vi "PH_Timing.PC Timing Mode.vi"(0 "i ref in":refnum<vi>, 2 "Timing Mode":T1 {"T2" min=0 max=6000 step=2}, 5 "error IO":errorcluster) -> (14 "i ref out":refnum<vi>, 19 "error out":errorcluster)   [LabVIEW 2014, in "PH_Timing.lvlib"]
doc: "This is a certain process case of Timing."
uses:
  PH_Timing.lvlib
  PH_Timing.Timing Mode.ctl
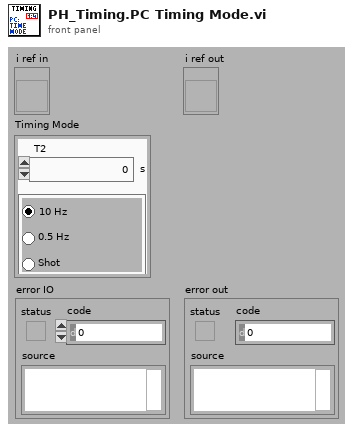
[diagram p1: front panel]
types:
  T1 = typedef "PH_Timing.lvlib/PH_Timing.Timing Mode.ctl" = cluster{"T2":i16, "Modeselector":enum32{"10 Hz", "0.5 Hz", "Shot"}}
  T2 = typedef "PH_Timing.lvlib/PH_Timing.i attribute.ctl" = cluster{"Sequencer":cluster{"linked?":bool, "Proc State":string, "Ref State":refnum<vi>}, "Gate Generator":cluster{"GD":cluster{"Device Status":T3, "linked?":bool}, "Settings":T4, "GUI Ref":refnum<vi>}, "Interlock Bypass":cluster{"Instancename":string, "Switch linked?":bool, "Device Status":T3, "Ref Status":refnum<vi>}, "Roughtuner":cluster{"Settings":T5, "GUI Ref":refnum<vi>, "GD":cluster{"Device Status":T3, "linked?":bool}}, "0,5Hz Gater":cluster{"Settings":T6, "GUI Ref":refnum<vi>, "GD":cluster{"Device Status":T3, "linked?":bool}}, "Slow Trigger":cluster{"Settings":T7, "GUI Ref":refnum<vi>, "Service ID Delay":i32, "Service ID Ext Trig":i32, "Wanted Settings":T7}, "Timing Mode":cluster{"Mode":T1, "GUI Ref":refnum<vi>, "Service ID T2":i32, "Service ID Mode":i32, "Wanted Mode":T1}, "ns Generator":cluster{"Settings":T8, "ns Generator Settings":refnum<vi>, "GD":cluster{"Device Status":T3, "linked?":bool}}, "Phase FEs":cluster{"Settings":T11, "GUI Ref":refnum<vi>, "Service ID Phase":i32, "Wanted Settings":T11}, "GD GUI Refs":refnum<vi>[], "Heads":T12[], "GUI Ref Delete":refnum<vi>}
  T3 = typedef "PH_StatusHandler.lvlib/PH_StatusHandler.Status.ctl" = i16
  T4 = typedef "PH_Timing.lvlib/PH_Timing.GateGen.ctl" = cluster{"Instance":string, "Channel Gate":i32, "Channel T2":i32, "Width Gate":dbl, "Width T2":dbl, "Delay Gate":dbl, "Delay T2":dbl, "Gate activ":bool, "T2 activ":bool, "System Mode":enum16{"Normal", "Single", "Burst", "Duty Cycle"}}
  T5 = typedef "PH_Timing.lvlib/PH_Timing.Roughtuner.ctl" = cluster{"Instance":string, "Phase PHELIX / UNILAC":cluster{"Channel":u16, "relative to":u16, "Delay [ms]":dbl}, "Pulse Length":cluster{"Channel":u16, "relative to":u16, "Delay [ms]":dbl}, "Trigger":cluster{"externally?":bool, "Rate [Hz]":dbl}}
  T6 = typedef "PH_Timing.lvlib/PH_Timing.0.5HzGater.ctl" = cluster{"Instance":string, "Channel ns FE Delay":i32, "Channel 0.5Hz":i32, "Width ns FE Delay":dbl, "Width 0.5Hz":dbl, "Delay ns FE Delay":dbl, "Delay 0.5Hz":dbl, "ns FE Delay active":bool, "0.5Hz activ":bool, "ns FE Delay inverted":bool, "0.5Hz inverted":bool}
  T7 = typedef "PH_Timing.lvlib/PH_Timing.Slow Trigger Settings.ctl" = cluster{"Delay":dbl, "externally triggered?":bool}
  T8 = typedef "PH_Timing.lvlib/PH_Timing.ns Generator.ctl" = cluster{"Instance":string, "Phase fs / ns FE":cluster{"Channel":T9, "Settings":T10}}
  T9 = typedef "Stanford Research DG645 - Driver.lvlib/Channel.ctl" = i32
  T10 = typedef "PH_SRDG645.lvlib/PH_SRDG645.Channel Settings.ctl" = cluster{"Delay [s]":dbl, "relative to":i32}
  T11 = typedef "PH_Timing.lvlib/PH_Timing.Phase FEs.ctl" = cluster{"Phase":dbl}
  T12 = typedef "PH_Timing.lvlib/PH_Timing.PU Data.ctl" = cluster{"linked?":bool, "Data":T13, "GD":cluster{"Device Status":T3, "linked?":bool}, "GUI Ref":refnum<vi>, "PU":T14}
  T13 = typedef "PH_Timing.lvlib/PH_Timing.PU Info.ctl" = cluster{"Act CH?":bool, "GD":string, "CH":i32, "Delay":dbl, "active":bool, "in Use?":bool}
  T14 = typedef "PH_PP_Common.lvlib/PH_PP_Common.PUs.ctl" = enum16{"no Info", "PA-19mm-1", "PA-19mm-2", "PA-45mm-PILC", "PA-45mm-MAIN", "MA-PU-1", "MA-PU-2", "MA-PU-3", "MA-PU-4", "MA-PU-5", "MA-PU-6", "MA-FR", "MA-PILC", "PA-45mm-DP"}
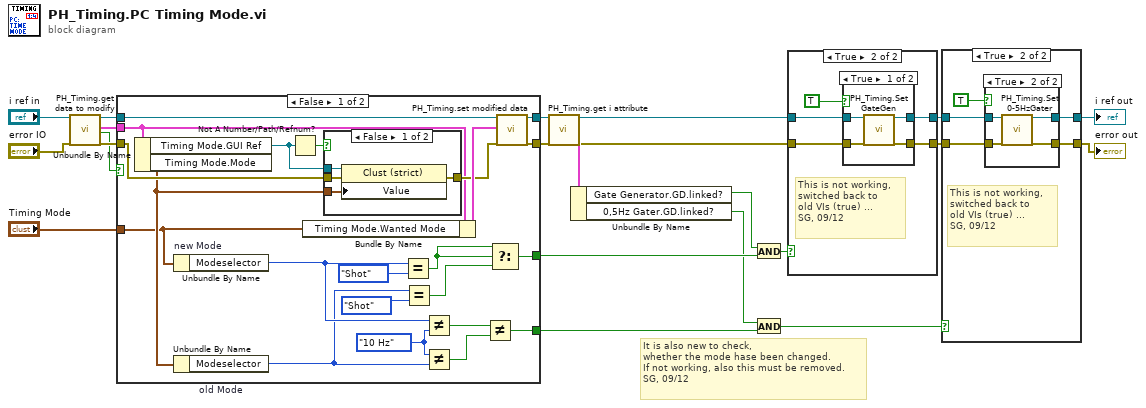
[diagram p0: block diagram]
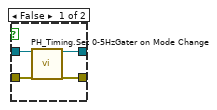
[diagram p3: hidden frame]
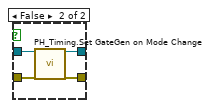
[diagram p5: hidden frame]
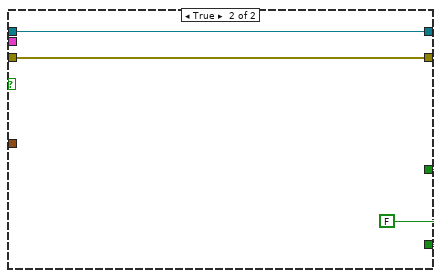
[diagram p7: hidden frame]
diagram:
  # "It is also new to check,\nwhether the mode hase been changed.\nIf not working, also this must be removed.\nSG, 09/12"
  n1 = call "PH_Timing.get data to modify.vi"("i ref in"="i ref in", "error in (no error)"="error IO") -> ("i ref out"=w22:refnum<vi>, "i attribute"=w20:T2, "timed out"=w19:bool, "error out"=w21:errorcluster)  [unwired: 14 in]
  n2 = case shown="False" w19 {
    tunnel: w22 -> [w44 w52]
    tunnel: [w43 w52] -> w13
    tunnel: w21 -> [w40 w51]
    tunnel: [w42 w51] -> w11
    tunnel: w20 -> [w30 _]
    tunnel: "Timing Mode" -> [w35 _]
    tunnel: [w32 w50] -> w6
    tunnel: [w25 w50] -> w5
    frame False {
      w31 = enum32{"10 Hz", "0.5 Hz", "Shot"}."10 Hz" ("Timing Mode.Wanted Mode.Modeselector")
      n3 = Unbundle By Name(w30) -> ("Timing Mode.GUI Ref"=w37:refnum<vi>, "Timing Mode.Mode"=w36:T1)
      n4 = Unbundle By Name "new Mode"(w35) -> ("Modeselector"=w29:enum32{"10 Hz", "0.5 Hz", "Shot"})
      n5 = Unbundle By Name "old Mode"(w36) -> ("Modeselector"=w26:enum32{"10 Hz", "0.5 Hz", "Shot"})
      n6 = Not A Number/Path/Refnum?(number/path/refnum=w37) -> (NaN/Path/Refnum?=w38:bool)
      n7 = Bundle By Name(cluster=w30, "Timing Mode.Wanted Mode"=w35) -> (w41:T2)
      n8 = case shown="False" w38 {
        tunnel: w37 -> [w48 _]
        tunnel: w36 -> [w47 _]
        tunnel: w40 -> [w46 w49]
        tunnel: [w45 w49] -> w39
        frame False {
          n9 = property class="Clust (strict)"(reference=w48, error in=w46, "Value"=w47) -> (error out=w45:errorcluster)  [unwired: 1 out]
        }
        frame True {
        }
      }
      n10 = Equal?(x=w29, y=enum32{"10 Hz", "0.5 Hz", "Shot"}."Shot") -> (x = y?=w23:bool)
      n11 = Equal?(x=w26, y=enum32{"10 Hz", "0.5 Hz", "Shot"}."Shot") -> (x = y?=w24:bool)
      n12 = Not Equal?(x=w29, y=w31) -> (x != y?=w34:bool)
      n13 = Not Equal?(x=w31, y=w26) -> (x != y?=w33:bool)
      n14 = Not Equal?(x=w34, y=w33) -> (x != y?=w32:bool)
      n15 = Select(t=w23, s=w23, f=w24) -> (s? t:f=w25:bool)
      n16 = call "PH_Timing.set modified data.vi"("i ref in"=w44, "i attribute"=w41, "error in (no error)"=w39) -> ("i ref out"=w43:refnum<vi>, "error out"=w42:errorcluster)  [unwired: 15 in]
    }
    frame True {
      w50 = FALSE
    }
  }
  n17 = call "PH_Timing.get i attribute.vi"("i ref in"=w13, "error in (no error)"=w11) -> ("i ref out"=w14:refnum<vi>, "i attribute"=w15:T2, "error out"=w12:errorcluster)  [unwired: 15 in]
  n18 = Unbundle By Name(w15) -> ("Gate Generator.GD.linked?"=w2:bool, "0,5Hz Gater.GD.linked?"=w1:bool)
  n19 = And(x=w2, y=w5) -> (x .and. y?=w3:bool)
  n20 = And(x=w1, y=w6) -> (x .and. y?=w4:bool)
  n21 = case shown="True" w3 {
    tunnel: [w54 w59] -> w9
    tunnel: [w53 w58] -> w7
    tunnel: w14 -> [w54 w57]
    tunnel: w12 -> [w53 w56]
    frame False {
    }
    frame True {
      # "This is not working, \nswitched back to\nold VIs (true) ...\nSG, 09/12"
      n22 = case shown="True" TRUE {
        tunnel: [w63 w67] -> w59
        tunnel: [w62 w66] -> w58
        tunnel: w57 -> [w61 w65]
        tunnel: w56 -> [w60 w64]
        frame True {
          n23 = call "PH_Timing.Set GateGen.vi"("i ref in"=w61, "error in (no error)"=w60) -> ("i ref out"=w63:refnum<vi>, "error out"=w62:errorcluster)  [unwired: 16 in]
        }
        frame False {
          n24 = call "PH_Timing.Set GateGen on Mode Change.vi"("i ref in"=w65, "error in (no error)"=w64) -> ("i ref out"=w67:refnum<vi>, "error out"=w66:errorcluster)  [unwired: 16 in]
        }
      }
    }
  }
  n25 = case shown="True" w4 {
    tunnel: [w69 w72] -> w10
    tunnel: w9 -> [w69 w74]
    tunnel: [w68 w71] -> w8
    tunnel: w7 -> [w68 w73]
    frame False {
    }
    frame True {
      # "This is not working, \nswitched back to\nold VIs (true) ...\nSG, 09/12"
      n26 = case shown="True" TRUE {
        tunnel: w74 -> [w78 w82]
        tunnel: w73 -> [w77 w81]
        tunnel: [w76 w80] -> w72
        tunnel: [w75 w79] -> w71
        frame False {
          n27 = call "PH_Timing.Set 0-5HzGater on Mode Change.vi"("i ref in"=w78, "error in"=w77) -> ("i ref out"=w76:refnum<vi>, "error out"=w75:errorcluster)  [unwired: 16 in]
        }
        frame True {
          n28 = call "PH_Timing.Set 0-5HzGater.vi"("i ref in"=w82, "error in (no error)"=w81) -> ("i ref out"=w80:refnum<vi>, "error out"=w79:errorcluster)  [unwired: 16 in]
        }
      }
    }
  }
  "i ref out" <- w10
  "error out" <- w8
